vi "Arduino Command Builder.vi"(8 "error in":errorcluster, 10 "Commands":string[](array[string]), 11 "Arduino in":refnum<visa-resource-name>) -> (0 "error out":errorcluster, 3 "Arduino out":refnum<visa-resource-name>)   [LabVIEW 2024]
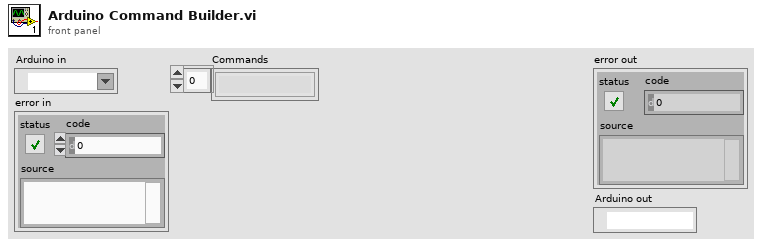
[diagram p1: front panel]
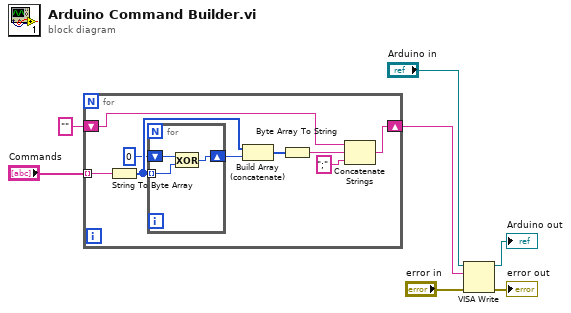
[diagram p0: block diagram]
diagram:
  n1 = for {
    tunnel: "Commands" -> [w16] mode=indexing
    shift-right: [w9] -> w1
    shift-left: "" ("string") -> [w11]
    n2 = String To Byte Array(string=w16) -> (unsigned byte array=w13:u8[])
    n3 = for {
      shift-right: [w18] -> w15
      shift-left: u8 0 -> [w19]
      tunnel: w13 -> [w17] mode=indexing
      n4 = Exclusive Or(1:w17, 2:w19) -> (0:w18:u8)
    }
    n5 = Build Array (concatenate)(w13, w15) -> (w14:u8[])
    n6 = Byte Array To String(unsigned byte array=w14) -> (string=w10:string)
    n7 = Concatenate Strings(w11, w10, ";" ("string")) -> (w9:string)
  }
  n8 = VISA Write(VISA resource name="Arduino in", write buffer=w1, error in (no error)="error in") -> (VISA resource name out=→"Arduino out":refnum<visa-resource-name>, error out=→"error out":errorcluster)  [unwired: 1 out]
